vi "FP parse the data - Copy.vi"(0 "Nav String":string="$,G,43,13,230,P,10,20,120,T,10,10,330,L,14,36,110,A,3,5,B,7,8,C,16,20,D,-1,-1,S,08,12,234\r", 1 "Tug":string="G") -> (2 "Buoy locations":cluster{"regular expression":string, i32, i32}[](array[cluster]), 3 "Tug Location":T1, 4 "Time":cluster{i32, i32, i32}, 5 "Valid?":bool)   [LabVIEW 2014]
doc: "This VI find the position of the tug whose letter was passed: X, Y and Heading.. The position values are positions are in pixel locations with 0,0 being at the top left, the heading is in degrees. It also finds the buoy locations and the time in hrs, min , secs."
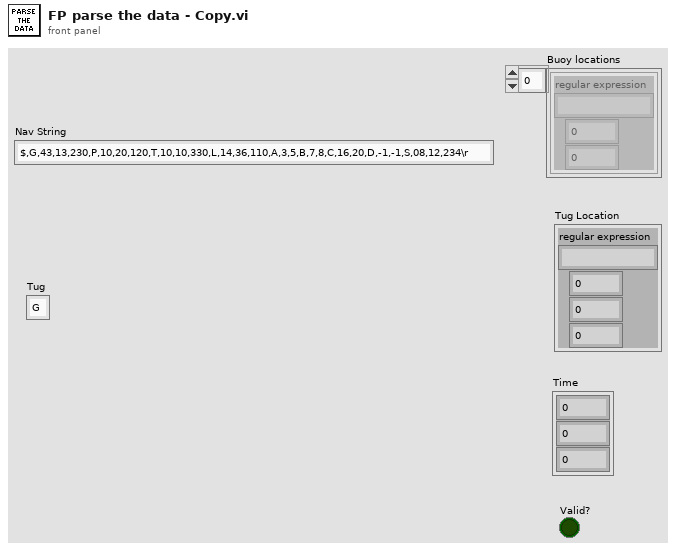
[diagram p1: front panel]
types:
  T1 = cluster{"regular expression":string, i32, i32, i32}
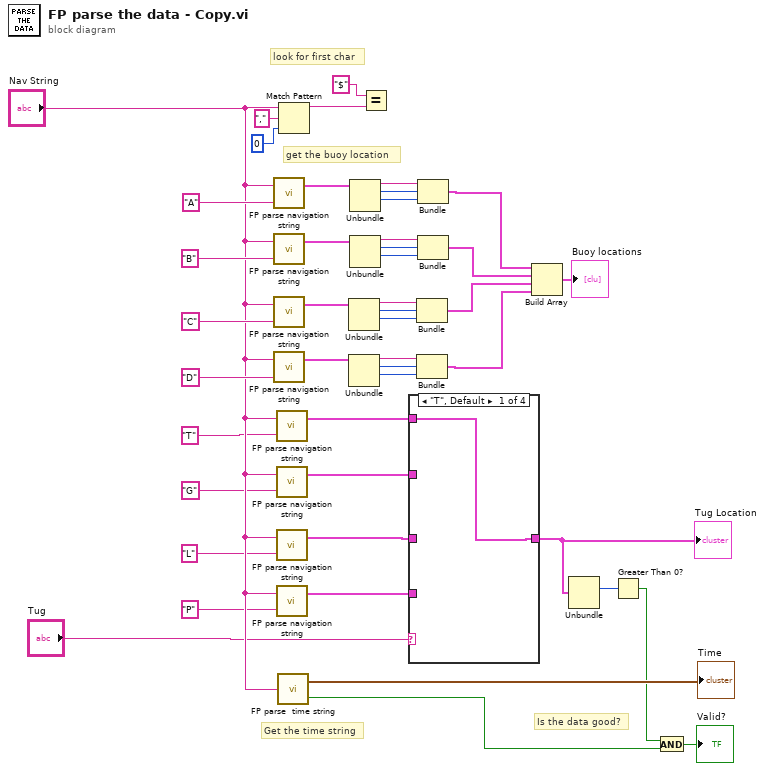
[diagram p0: block diagram]
diagram:
  # "Is the data good?"
  # "get the buoy location"
  # "Get the time string"
  # "look for first char"
  n1 = call "FP parse navigation string.vi"("Header"="A" ("Tug"), "Nav String"="Nav String") -> ("Nav Data"=w40:T1)  [unwired: 1 out]
  n2 = call "FP parse navigation string.vi"("Header"="B" ("Tug"), "Nav String"="Nav String") -> ("Nav Data"=w35:T1)  [unwired: 1 out]
  n3 = call "FP parse navigation string.vi"("Header"="C" ("Tug"), "Nav String"="Nav String") -> ("Nav Data"=w30:T1)  [unwired: 1 out]
  n4 = call "FP parse navigation string.vi"("Header"="D" ("Tug"), "Nav String"="Nav String") -> ("Nav Data"=w25:T1)  [unwired: 1 out]
  n5 = call "FP parse navigation string.vi"("Header"="T", "Nav String"="Nav String") -> ("Nav Data"=w10:T1)  [unwired: 1 out]
  n6 = call "FP parse navigation string.vi"("Header"="G", "Nav String"="Nav String") -> ("Nav Data"=w9:T1)  [unwired: 1 out]
  n7 = call "FP parse navigation string.vi"("Header"="L", "Nav String"="Nav String") -> ("Nav Data"=w7:T1)  [unwired: 1 out]
  n8 = call "FP parse navigation string.vi"("Header"="P", "Nav String"="Nav String") -> ("Nav Data"=w6:T1)  [unwired: 1 out]
  n9 = call "FP parse  time string.vi"("Nav String"="Nav String") -> ("output cluster"=→"Time":cluster{i32, i32, i32}, "Valid?"=w2:bool)
  n10 = Match Pattern(string="Nav String", regular expression=",", offset (0)=0) -> (before substring=w44:string)  [unwired: 3 out]
  n11 = Unbundle(w30) -> ("regular expression"=w29:string, w28:i32, w27:i32)  [unwired: 1 out]
  n12 = Unbundle(w25) -> ("regular expression"=w24:string, w23:i32, w22:i32)  [unwired: 1 out]
  n13 = Unbundle(w40) -> ("regular expression"=w39:string, w38:i32, w37:i32)  [unwired: 1 out]
  n14 = Unbundle(w35) -> ("regular expression"=w34:string, w33:i32, w32:i32)  [unwired: 1 out]
  n15 = Equal?(x="$", y=w44) -> ()  [unwired: 1 out]
  n16 = case shown="\"T\", Default" "Tug" {
    tunnel: w10 -> [w46 _ _ _]
    tunnel: w9 -> [_ w47 _ _]
    tunnel: w7 -> [_ _ w48 _]
    tunnel: w6 -> [_ _ _ w49]
    tunnel: [w46 w47 w48 w49] -> w5
    frame "T", Default {
    }
    frame "G" {
    }
    frame "L" {
    }
    frame "P" {
    }
  }
  "Tug Location" <- w5
  n17 = Bundle("regular expression"=w29, w28, w27) -> (w19:cluster{"regular expression":string, i32, i32})  [unwired: 1 in]
  n18 = Bundle("regular expression"=w24, w23, w22) -> (w18:cluster{"regular expression":string, i32, i32})  [unwired: 1 in]
  n19 = Bundle("regular expression"=w39, w38, w37) -> (w21:cluster{"regular expression":string, i32, i32})  [unwired: 1 in]
  n20 = Bundle("regular expression"=w34, w33, w32) -> (w20:cluster{"regular expression":string, i32, i32})  [unwired: 1 in]
  n21 = Build Array(w21, w20, w19, w18) -> (→"Buoy locations":cluster{"regular expression":string, i32, i32}[])
  n22 = Unbundle(w5) -> (w4:i32)  [unwired: 3 out]
  n23 = Greater Than 0?(x=w4) -> (x > 0?=w1:bool)
  n24 = And(x=w1, y=w2) -> (x .and. y?=→"Valid?":bool)
